vi "Read Command to Execute.vi"(8 "error in (no error)":errorcluster, 11 "User Defined Read in":refnum<class "User Defined Read.lvclass">) -> (0 "error out":errorcluster, 2 "Command to Execute":string, 3 "User Defined Read out":refnum<class "User Defined Read.lvclass">)   [LabVIEW 2023, in "HAF.lvlib" / "User Defined Read.lvclass"]
doc: "Returns the SCPI command that this Command is responsible for running."
uses:
  User Defined Read.lvclass
  User Defined Read.lvclass/User Defined Read.ctl
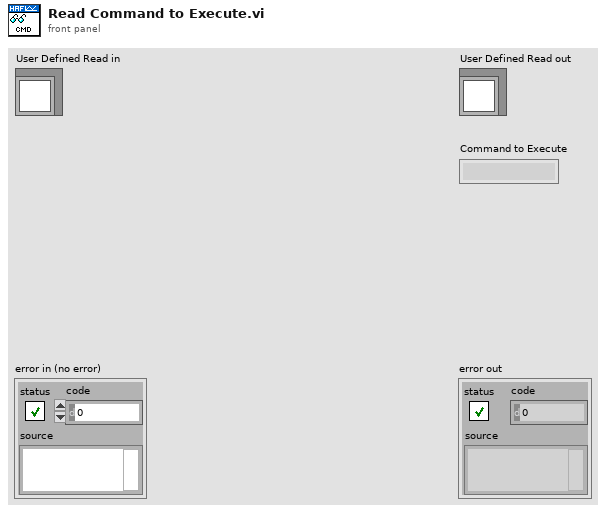
[diagram p1: front panel]
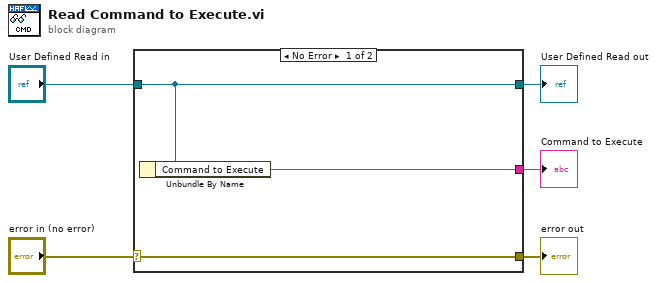
[diagram p0: block diagram]
diagram:
  n1 = case shown="No Error" "error in (no error)" {
    selector: "error in (no error)" -> [w8 w9]
    tunnel: [w8 w9] -> w4
    tunnel: [w7 w10] -> w2
    tunnel: "User Defined Read in" -> [w7 w10]
    tunnel: [w6 _] -> w1
    frame No Error {
      n2 = Unbundle By Name(w7) -> ("Command to Execute"=w6:string)
    }
    frame Error {
    }
  }
  "error out" <- w4
  "User Defined Read out" <- w2
  "Command to Execute" <- w1
